vi "多参数报警信息.vi"(8 "error in (no error)":errorcluster, 11 "data":T1) -> (0 "error out":errorcluster)   [LabVIEW 2016, in "斯坦道原位多参数.lvlib"]
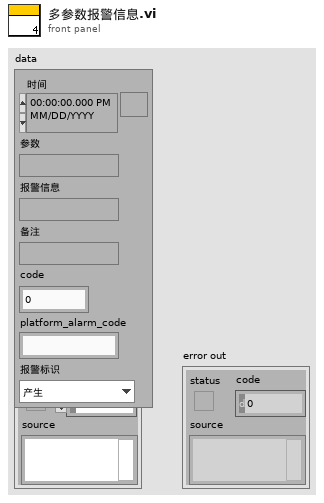
[diagram p1: front panel]
types:
  T1 = typedef "报警信息字段定义.ctl" = cluster{"时间":timestamp, "参数":string, "报警信息":string, "备注":string, "code":u64, "platform_alarm_code":string, "报警标识":enum16{"产生", "消除"}}
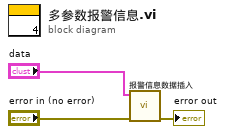
[diagram p0: block diagram]
diagram:
  n1 = call "报警信息数据插入.vi"("data"="data", "错误输入（无错误）"="error in (no error)") -> ("错误输出"=→"error out":errorcluster)  [unwired: 8 in]
